vi "ListboxCreate.vi"(0 "HP34401 input":dbl format="%#_5f", 2 "Current B":dbl(knob) caption="I [mA]" min=0.0 max=50.0 step=0.01 scale=0.0..50.0 scale format="%#.3f", 3 "Current  A":dbl(knob) caption="I [mA]" min=0.0 max=50.0 step=0.01 scale=0.0..50.0 scale format="%#.3f", 5 "Array input":string[][](array[string])) -> (1 "Array output":string[][](array[string]))   [LabVIEW 2021]
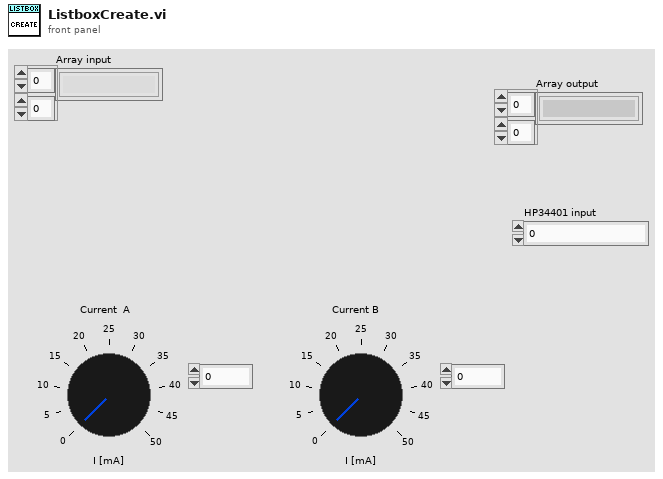
[diagram p1: front panel]
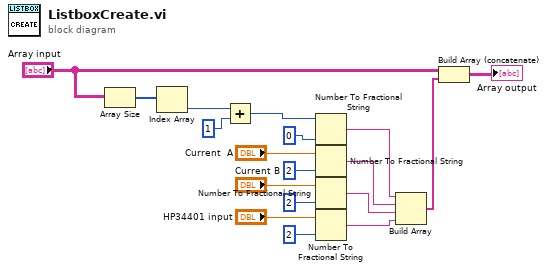
[diagram p0: block diagram]
diagram:
  n1 = Array Size(array="Array input") -> (size(s)=w18:i32[])
  n2 = Index Array(array=w18) -> (element=w13:i32)  [unwired: 1 in]
  n3 = Add(x=w13, y=1) -> (x+y=w12:i32)
  n4 = Number To Fractional String(number=w12, precision (6)=i16 0) -> (F-format string=w15:string)  [unwired: 2 in]
  n5 = Number To Fractional String(number="Current  A", precision (6)=i16 2) -> (F-format string=w17:string)  [unwired: 2 in]
  n6 = Number To Fractional String(number="Current B", precision (6)=i16 2) -> (F-format string=w16:string)  [unwired: 2 in]
  n7 = Number To Fractional String(number="HP34401 input", precision (6)=i16 2) -> (F-format string=w7:string)  [unwired: 2 in]
  n8 = Build Array(w15, w17, w16, w7) -> (w10:string[])
  n9 = Build Array (concatenate)("Array input", w10) -> (→"Array output":string[][])
